vi "System@ExternalDeviceCMD__Parameter.vi"(1 "ParamterIn":string) -> (0 "ParamterOut":string)   [LabVIEW 2019]
panel:
  in  "Parameter":string(combo)
  in  "CMD":string(combo)
  in  "Device":string(combo)
  in  "Confirm":bool
  # "System@ExternalDeviceCMD $DeviceName,$Command,$Parameter"
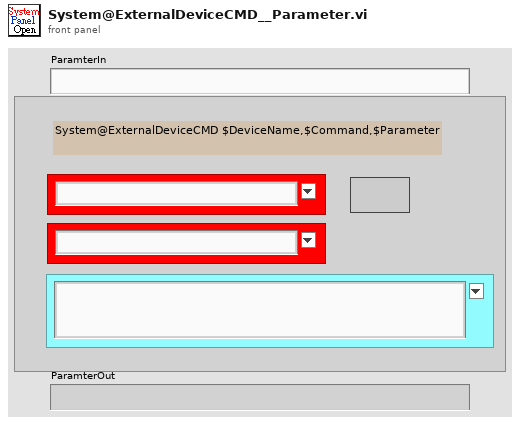
[diagram p1: front panel]
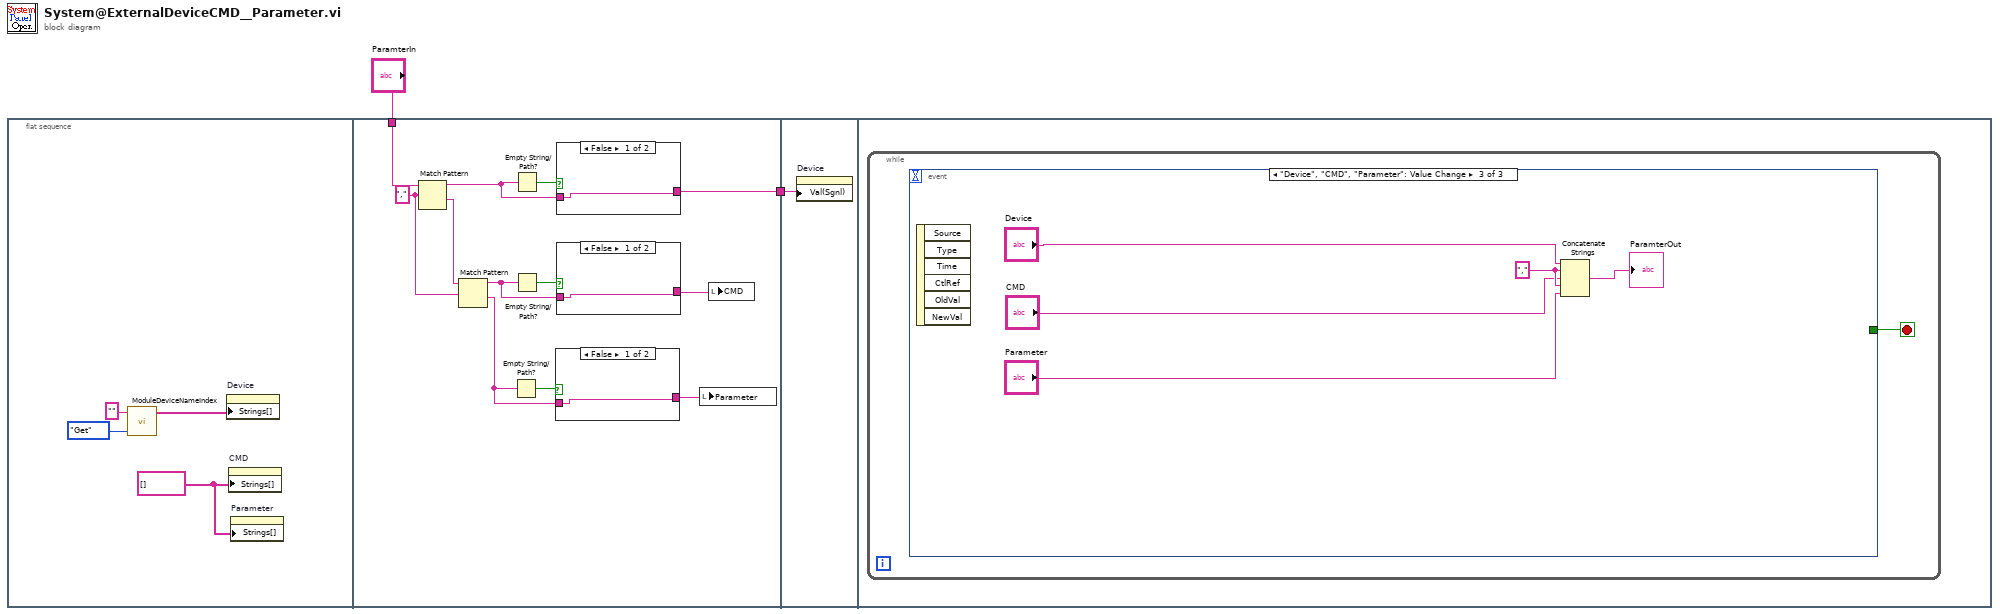
[diagram p0: block diagram]
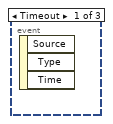
[diagram p5: hidden frame]
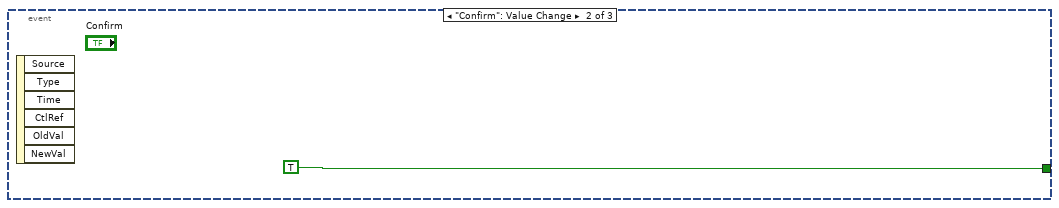
[diagram p6: hidden frame]
diagram:
  n1 = flat-sequence {
    tunnel: "ParamterIn" -> [w16]
    tunnel: [w17] -> w1
    tunnel: w1 -> [w25]
    frame #0 {
      w3 = string[] [] ("Strings []")
      n2 = call "ModuleDeviceNameIndex.vi"("OP"=enum16{"Get", "Update", "Init"}."Get", "DeviceName"="") -> ("DeviceList"=w4:string[])  [unwired: 1 in, 2 out]
      n3 = property on="Device" class="CmbBox"("Strings[]"=w4) -> ()  [unwired: 2 in, 2 out]
      n4 = property on="CMD" class="CmbBox"("Strings[]"=w3) -> ()  [unwired: 2 in, 2 out]
      n5 = property on="Parameter" class="CmbBox"("Strings[]"=w3) -> ()  [unwired: 2 in, 2 out]
    }
    frame #1 {
      w12 = "," ("regular expression")
      n6 = Match Pattern(string=w16, regular expression=w12) -> (before substring=w14:string, after substring=w11:string)  [unwired: 1 in, 2 out]
      n7 = Match Pattern(string=w11, regular expression=w12) -> (before substring=w10:string, after substring=w8:string)  [unwired: 1 in, 2 out]
      n8 = Empty String/Path?(string/path=w8) -> (empty?=w9:bool)
      n9 = Empty String/Path?(string/path=w14) -> (empty?=w18:bool)
      n10 = Empty String/Path?(string/path=w10) -> (empty?=w15:bool)
      n11 = case shown="False" w9 {
        tunnel: w8 -> [w19 w20]
        tunnel: [w19 w20] -> w7
        frame False {
        }
        frame True {
        }
      }
      n12 = case shown="False" w18 {
        tunnel: w14 -> [w23 w24]
        tunnel: [w23 w24] -> w17
        frame False {
        }
        frame True {
        }
      }
      n13 = case shown="False" w15 {
        tunnel: w10 -> [w21 w22]
        tunnel: [w21 w22] -> w13
        frame False {
        }
        frame True {
        }
      }
      n14 = local write "Parameter"(w7) -> ()
      n15 = local write "CMD"(w13) -> ()
    }
    frame #2 {
      n16 = property on="Device" class="CmbBox"("Val(Sgnl)"=w25) -> ()  [unwired: 2 in, 2 out]
    }
    frame #3 {
      n17 = while {
        stop <- w26 stop-if-true
        n18 = event shown="[2] \"Device\", \"CMD\", \"Parameter\": Value Change" {
          selector: _ -> [_ _ _]
          dyn-events: _ -> [_ _ _]
          timeout: _ -> [_ _ _]
          tunnel: [_ TRUE _] -> w26
          event Timeout {
            n19 = event-data() -> ()  [unwired: 1 in, 3 out]
          }
          event "Confirm": Value Change {
            n20 = event-data() -> ()  [unwired: 1 in, 6 out]
          }
          event "Device", "CMD", "Parameter": Value Change {
            w30 = "," ("string")
            n21 = event-data() -> ()  [unwired: 1 in, 6 out]
            n22 = Concatenate Strings("Device", w30, "CMD", w30, "Parameter") -> (→"ParamterOut":string)
          }
        }
      }
    }
  }
